vi "GetOpcode.vi"(9 "Byte Packet in":u8) -> (1 "Opcode":T1, 2 "Byte Packet out":u8)   [LabVIEW 2016, in "WebSockets.lvlib"]
uses:
  WebSockets.lvlib
  Opcode.ctl
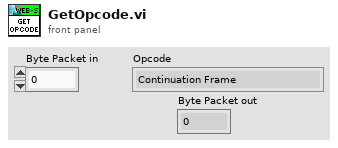
[diagram p1: front panel]
types:
  T1 = typedef "WebSockets.lvlib/Opcode.ctl" = enum8{"Continuation Frame", "Text Frame", "Binary Frame", "Reserved 3", "Reserved 4", "Reserved 5", "Reserved 6", "Reserved 7", "Connection Close", "Ping", "Pong", "Reserved B", "Reserved C", "Reserved D", "Reserved F"}
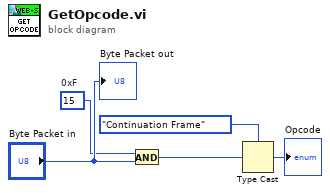
[diagram p0: block diagram]
diagram:
  w4 = u8 15  # 0xF
  n1 = And(x=w4, y="Byte Packet in") -> (x .and. y?=w1:u8)
  n2 = Type Cast(type=Opcode."Continuation Frame" ("Opcode"), x=w1) -> (*(type *) &x=→"Opcode":T1)
  "Byte Packet out" <- "Byte Packet in"
